vi "errorNumberToString.vi"(8 "error":errorcluster, 9 "errNbr":i32, 10 "language":i32, 11 "connection ID":refnum<k5>) -> (0 "error out":errorcluster, 2 "message":string, 3 "connection ID out":refnum<k5>)   [LabVIEW 2016, in "amc_api.lvlib"]
doc: "Gets a description of an error code."
uses:
  amc_api.lvlib
panel:
  out "jsonRespIn":string
  out "JSON-response":string="{\"jsonrpc\":\"2.0\",\"method\":\"\",\"params\":[5,1.245,true,\"name\"],\"id\":\"1\"}"
  out "JSON request":string
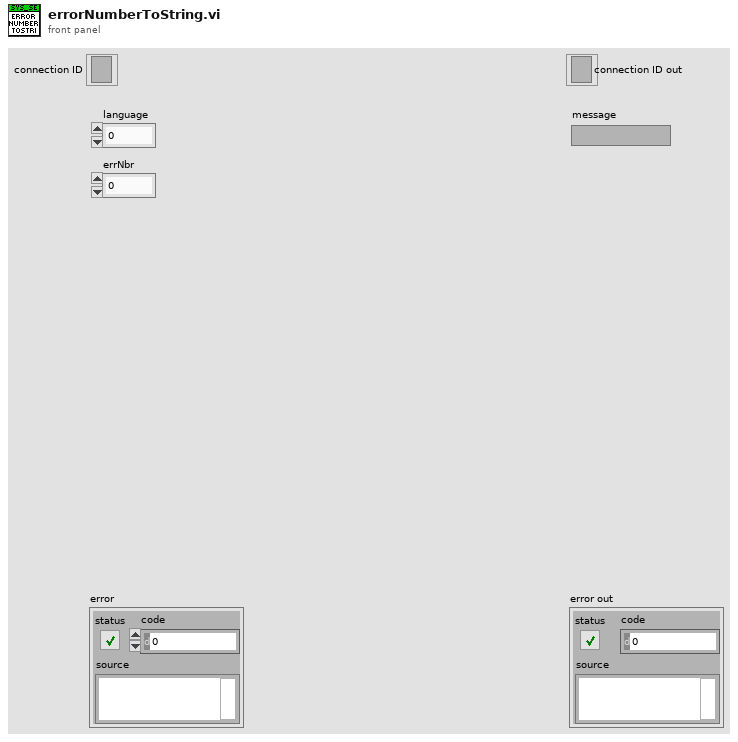
[diagram p1: front panel]
types:
  T1 = cluster{"jsonrpc":string, "method":string, "params":string[], "id":string, "api":i32, "pid":string}
  T2 = enum16{"Standard", "Buffered", "CRLF", "Immediate"}
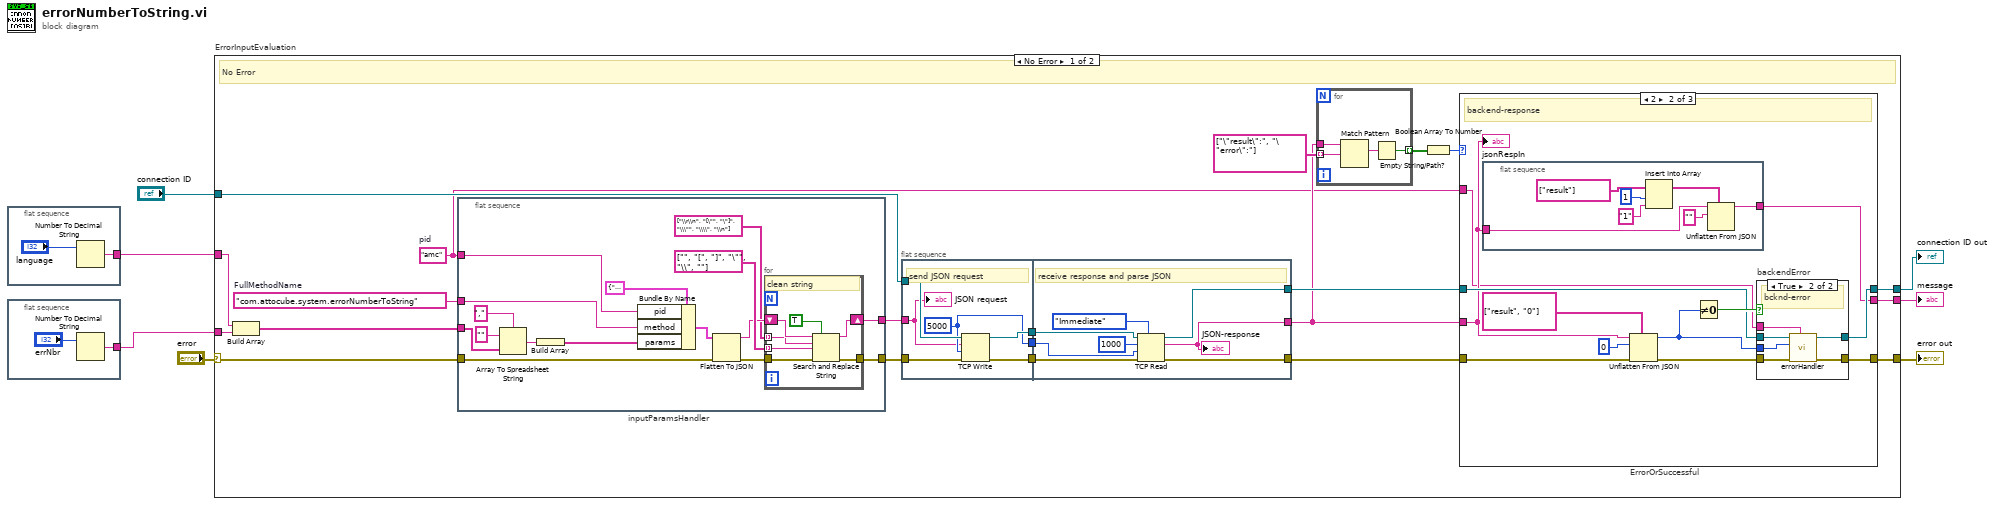
[diagram p0: block diagram]
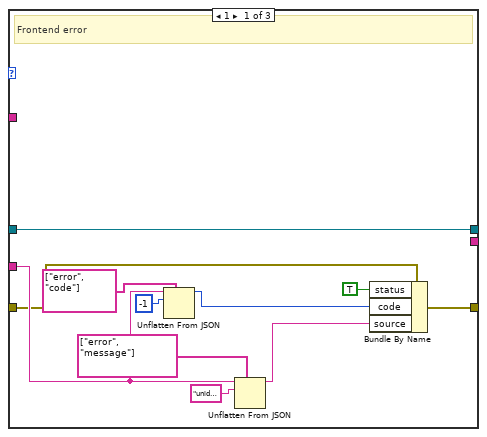
[diagram p2: hidden frame]
diagram:
  n1 = flat-sequence "in_integer" {
    tunnel: [w8] -> w3
    frame #0 {
      n2 = Number To Decimal String(number="language") -> (decimal integer string=w8:string)  [unwired: 1 in]
    }
  }
  n3 = flat-sequence "in_integer" {
    tunnel: [w10] -> w2
    frame #0 {
      n4 = Number To Decimal String(number="errNbr") -> (decimal integer string=w10:string)  [unwired: 1 in]
    }
  }
  n5 = case "ErrorInputEvaluation" shown="No Error" "error" {
    selector: "error" -> [w19 w114]
    tunnel: "connection ID" -> [w29 w115]
    tunnel: [w21 w114] -> w6
    tunnel: [w22 w115] -> w5
    tunnel: w3 -> [w14 _]
    tunnel: w2 -> [w13 _]
    tunnel: [w12 _] -> w1
    frame No Error {
      w15 = "amc"  # pid
      w20 = "com.attocube.system.errorNumberToString"  # FullMethodName
      # "No Error"
      n6 = Build Array ("ParametersArrayString")(w14, w13) -> (w18:string[])
      n7 = flat-sequence "inputParamsHandler" {
        tunnel: [w38] -> w17
        tunnel: w18 -> [w44]
        tunnel: w19 -> [w43]
        tunnel: [w40] -> w16
        tunnel: w20 -> [w34]
        tunnel: w15 -> [w33]
        frame #0 {
          n8 = Array To Spreadsheet String(delimiter (Tab)=",", array=w44, 3:"" ("format string")) -> (spreadsheet string=w46:string)
          n9 = Build Array "Build Array"(w46) -> (w35:string[])
          n10 = Bundle By Name(cluster=T1 {"jsonrpc"="2.0", "method"="com.attocube.amc.res.setRESReadOutFreq", "params"=[], "id"="1", "api"=2, "pid"=""}, "pid"=w33, "method"=w34, "params"=w35) -> (w45:T1)
          n11 = Flatten To JSON(anything=w45, error in (no error)=w43) -> (JSON string=w39:string, 11:w41:errorcluster)  [unwired: 1 in]
          n12 = for {
            tunnel: string[] ["\\r\\n", "[\"", "\"]", "\\\"", "\\\\", "\\n"] ("search string") -> [w52] mode=indexing
            tunnel: string[] ["", "[", "]", "\"", "\\", ""] ("replace string (\"\")") -> [w51] mode=indexing
            shift-right: [w54] -> w38
            shift-left: w39 -> [w53]
            tunnel: w41 -> [w50]
            tunnel: [w49] -> w40
            # "clean string"
            n13 = Search and Replace String(replace all?=TRUE ("replace all? (F)"), input string=w53, search string=w52, replace string=w51, error in=w50) -> (result string=w54:string, error out=w49:errorcluster)  [unwired: 3 in, 2 out]
          }
        }
      }
      n14 = flat-sequence {
        tunnel: w29 -> [w105]
        tunnel: [w103] -> w32
        tunnel: [w104] -> w31
        tunnel: w16 -> [w100]
        tunnel: [w102] -> w30
        tunnel: w17 -> [w101]
        tunnel: [w109] -> w25
        tunnel: w32 -> [w111]
        tunnel: w31 -> [w110]
        tunnel: [w107] -> w24
        tunnel: w30 -> [w108]
        tunnel: [w106] -> w23
        frame #0 {
          w102 = 5000 ("timeout ms (25000)")
          # "send JSON request"
          n15 = TCP Write(connection ID=w105, data in=w101, error in (no error)=w100, 9:w102) -> (connection ID out=w103:refnum<k5>, error out=w104:errorcluster)  [unwired: 1 out]
          "JSON request" <- w101
        }
        frame #1 {
          # "receive response and parse JSON"
          n16 = TCP Read(connection ID=w111, bytes to read=1000, error in (no error)=w110, 7:T2."Immediate" ("mode (standard)"), 9:w108) -> (connection ID out=w109:refnum<k5>, data out=w106:string, error out=w107:errorcluster)
          "JSON-response" <- w106
        }
      }
      n17 = for {
        tunnel: string[] ["\"result\":", "\"error\":"] ("path") -> [w58] mode=indexing
        tunnel: [w56] -> w27 mode=indexing
        tunnel: w23 -> [w59]
        n18 = Match Pattern(string=w59, regular expression=w58) -> (match substring=w57:string)  [unwired: 1 in, 3 out]
        n19 = Empty String/Path?(string/path=w57) -> (empty?=w56:bool)
      }
      n20 = Boolean Array To Number(Boolean array=w27) -> (number=w26:u32)
      n21 = case "ErrorOrSuccessful" shown="2" w26 {
        tunnel: w23 -> [w62 w73 _]
        tunnel: w25 -> [w60 w76 w99]
        tunnel: [w60 w75 w99] -> w22
        tunnel: [w63 w74 w98] -> w21
        tunnel: w24 -> [w61 w77 w98]
        tunnel: w15 -> [_ w72 _]
        tunnel: [_ w71 _] -> w12
        frame 1 {
          # "Frontend error"
          n22 = Unflatten From JSON(path=string[] ["error", "code"], JSON string=w62, type and defaults=-1) -> (value=w69:i32)  [unwired: 4 in, 1 out]
          n23 = Unflatten From JSON(path=string[] ["error", "message"], JSON string=w62, type and defaults="unidentified error") -> (value=w70:string)  [unwired: 4 in, 1 out]
          n24 = Bundle By Name(cluster=w61, "status"=TRUE, "code"=w69, "source"=w70) -> (w63:errorcluster)
        }
        frame 2 {
          # "backend-response"
          n25 = flat-sequence "out_string" {
            tunnel: w73 -> [w89]
            tunnel: [w83] -> w71
            frame #0 {
              n26 = Insert Into Array(array=string[] ["result"] ("path"), index=1, new element="1" ("idx")) -> (w86:string[])
              n27 = Unflatten From JSON(path=w86, JSON string=w89, type and defaults="") -> (value=w83:string)  [unwired: 4 in, 1 out]
            }
          }
          n28 = Unflatten From JSON(path=string[] ["result", "0"], JSON string=w73, type and defaults=0, error in (no error)=w77) -> (value=w82:i32, error out=w80:errorcluster)  [unwired: 3 in]
          n29 = Not Equal To 0?(x=w82) -> (x != 0?=w81:bool)
          n30 = case "backendError" shown="True" w81 {
            tunnel: w82 -> [_ w97]
            tunnel: w80 -> [w91 w96]
            tunnel: [w90 w95] -> w75
            tunnel: [w91 w94] -> w74
            tunnel: w76 -> [w90 w93]
            tunnel: w72 -> [_ w92]
            frame False {
              # "successful"
            }
            frame True {
              # "bcknd-error"
              n31 = call "errorHandler.vi"("pid"=w92, "error in"=w96, "errNbr"=w97, "connection ID"=w93) -> ("error out 2"=w94:errorcluster, "connection ID out"=w95:refnum<k5>)  [unwired: 6 in]
            }
          }
          "jsonRespIn" <- w73
        }
        frame Default {
          # "NoResponse"
        }
      }
    }
    frame Error {
      # "Error"
    }
  }
  "error out" <- w6
  "connection ID out" <- w5
  "message" <- w1
